vi "VisibleTabControlPage.vi"() -> ()   [LabVIEW 2014]
doc: "This example shows how to make a single tab control page visible and hide all other pages without the pages appearing grayed. Using Property Nodes alone might result in grayed pages, because the Property Node hides the current page and grays it before it makes another page visible. You can use an Event structure to make a page visible and make it the current page before hiding all other pages."
panel:
  in  "First Tab Control":enum32{"Page 1", "Page 2", "Page 3"}(tab) caption="Method that Can Result in Grayed Pages"
  out "Boolean 3":bool
  in  "Slide 2":dbl(slide) scale=0.0..10.0
  out "Gauge 2":dbl(knob) scale=0.0..10.0
  in  "Stop":bool
  in  "Cluster":T1
  in  "Second Tab Control":enum32{"Page 1", "Page 2", "Page 3"}(tab)=enum."Page 3" caption="Method that Results in No Grayed Pages"
  out "Boolean 2":bool
  in  "Slide":dbl(slide) scale=0.0..10.0
  out "Gauge":dbl(knob) scale=0.0..10.0
  # "Visible?"
  # "Click a button to make that tab control\npage visible and hide all other pages.\n\nIf you click several buttons you will notice\ngrayed pages in the first method."
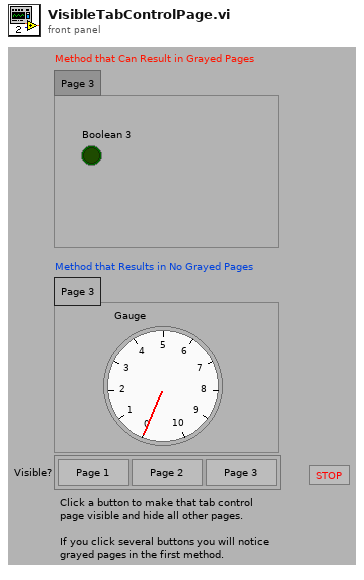
[diagram p1: front panel]
types:
  T1 = cluster{"OK Button":bool, "OK Button 2":bool, "OK Button 3":bool}
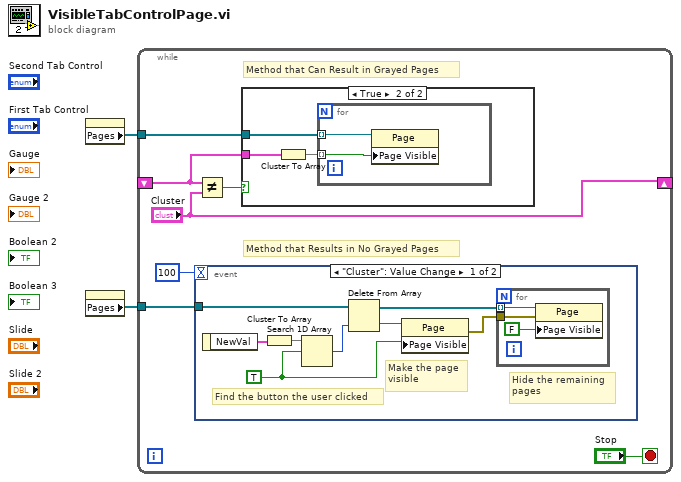
[diagram p0: block diagram]
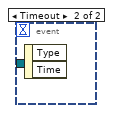
[diagram p3: hidden frame]
diagram:
  n1 = property on="First Tab Control" class="TabCtl (strict)"() -> ("Pages"=w1:refnum<vi>[])  [unwired: 2 in, 2 out]
  n2 = property on="Second Tab Control" class="TabCtl (strict)"() -> ("Pages"=w2:refnum<vi>[])  [unwired: 2 in, 2 out]
  n3 = while {
    tunnel: w2 -> [w7]
    tunnel: w1 -> [w6]
    shift-right: ["Cluster"] -> _
    shift-left: _ -> [w3]
    stop <- "Stop" stop-if-true
    # "Method that Results in No Grayed Pages"
    # "Method that Can Result in Grayed Pages"
    n4 = event shown="[0] \"Cluster\": Value Change" {
      selector: _ -> [_ _]
      dyn-events: _ -> [_ _]
      timeout: 100 -> [_ _]
      tunnel: w7 -> [w15 _]
      event "Cluster": Value Change {
        w20 = TRUE ("element")
        # "Find the button the user clicked"
        # "Hide the remaining\npages"
        # "Make the page\nvisible"
        n5 = event-data() -> ("NewVal"=w22:T1)  [unwired: 1 in]
        n6 = Cluster To Array(cluster=w22) -> (array=w21:bool[])
        n7 = Search 1D Array(1D array=w21, element=w20) -> (index of element=w19:i32)  [unwired: 1 in]
        n8 = Delete From Array(array=w15, index=w19) -> (deleted portion=w18:refnum<vi>, array with subset deleted=w17:refnum<vi>[])  [unwired: 1 in]
        n9 = property class="Page"(reference=w18, "Page Visible"=w20) -> (error out=w16:errorcluster)  [unwired: 1 in, 1 out]
        n10 = for {
          tunnel: w17 -> [w25] mode=indexing
          tunnel: w16 -> [w24]
          n11 = property class="Page"(reference=w25, error in=w24, "Page Visible"=FALSE) -> ()  [unwired: 2 out]
        }
      }
      event Timeout {
        n12 = event-data() -> ()  [unwired: 1 in, 2 out]
      }
    }
    n13 = Not Equal?(x=w3, y="Cluster") -> (x != y?=w5:bool)
    n14 = case shown="True" w5 {
      tunnel: w6 -> [_ w12]
      tunnel: w3 -> [_ w10]
      frame False {
      }
      frame True {
        n15 = Cluster To Array(cluster=w10) -> (array=w11:bool[])
        n16 = for {
          tunnel: w12 -> [w14] mode=indexing
          tunnel: w11 -> [w13] mode=indexing
          n17 = property class="Page"(reference=w14, "Page Visible"=w13) -> ()  [unwired: 1 in, 2 out]
        }
      }
    }
  }
